vi "destroy.vi"(8 "error in (no error)":errorcluster, 11 "json.provider in":refnum<class "json.provider.lvclass">) -> (0 "error out":errorcluster)   [LabVIEW 2021, in "json.provider.lvclass"]
uses:
  json.provider.lvclass
  json.provider.lvclass/json.provider.ctl
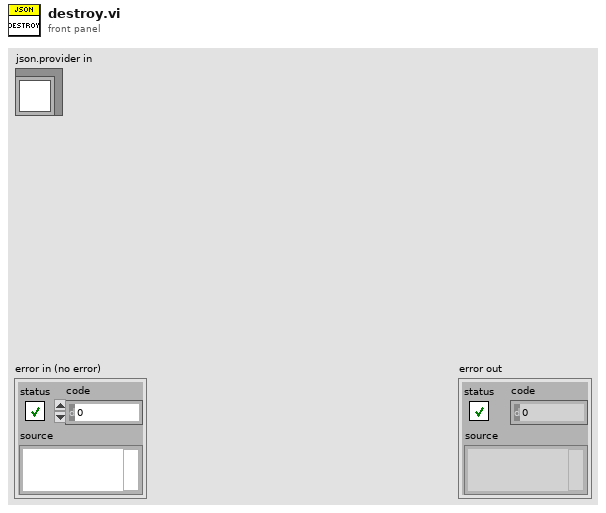
[diagram p1: front panel]
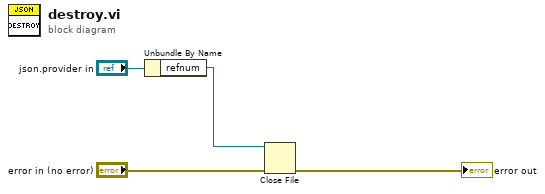
[diagram p0: block diagram]
diagram:
  n1 = Unbundle By Name("json.provider in") -> ("refnum"=w2:refnum<file>)
  n2 = Close File(refnum=w2, error in="error in (no error)") -> (error out=→"error out":errorcluster)  [unwired: 1 out]
